vi "Moving average filter.vi"(8 "x":i32, 11 "Input":i32) -> (0 "xdot":i32, 3 "Mean":i32)   [LabVIEW 2016]
doc: "Input\nRawdata\n\nOutput\nFiltered data\n\nCalculates the moving average of the data with a window size of 8."
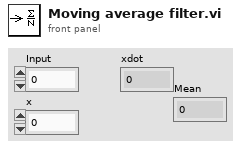
[diagram p1: front panel]
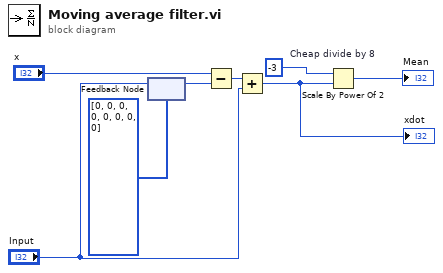
[diagram p0: block diagram]
diagram:
  n1 = feedback #1(i32[] [0, 0, 0, 0, 0, 0, 0, 0]) -> (w6:i32)
  n2 = feedback-in #1("Input") -> ()
  n3 = Subtract(x="x", y=w6) -> (x-y=w5:i32)
  n4 = Add(x=w5, y="Input") -> (x+y=w3:i32)
  "xdot" <- w3
  n5 = Scale By Power Of 2 "Cheap divide by 8"(n=i16 -3, x=w3) -> (x*2^n=→"Mean":i32)
